vi "LIA_FPGA3a-PD Test-3.vi"() -> (1 "K Constant":fxp<+/-,32,16>, 2 "Nominal Freq":fxp<+/-,64,32>)   [LabVIEW 2012]
uses:
  <vilib>/rvi/DataTransferAndStorage/Container/Common/niFpgaContainerMetaDataKey.ctl
  <vilib>/rvi/DataTransferAndStorage/Container/Common/niFpgaContainerState.ctl
  <vilib>/rvi/DataTransferAndStorage/Container/Common/niFpgaDataTypeControl.ctl
  <vilib>/rvi/DataTransferAndStorage/Container/Common/niFpgaContainerImplementationControl.ctl
  <vilib>/rvi/DataTransferAndStorage/Container/Common/niFpgaContainerArbitrationOptionsControl.ctl
  <vilib>/rvi/DataTransferAndStorage/Container/Common/niFpgaTransferTypeControl.ctl
  <vilib>/rvi/DataTransferAndStorage/Container/Common/niFpgaContainerInitializationParameters.ctl
  <vilib>/rvi/Memory/Memory_Types/niFpgaMemoryInterfaceConfiguration.ctl
  <vilib>/rvi/FIFO/Fifo_Types/niFpgaFifoControlLogicControl.ctl
  <vilib>/Platform/TimedLoop/XDataNode/timing_clust.ctl
  <vilib>/Platform/TimedLoop/XDataNode/nitl_modes.ctl
  <vilib>/Platform/TimedLoop/XDataNode/wakeup.ctl
  <vilib>/rvi/FXPMathLib/FxpSinAndCos/subVIs/nifxpmath_SinAndCos_SimConfig.ctl
  <vilib>/rvi/FXPMathLib/basic elements/FxpIntAccumulator/subVIs/nifxpmath_IntAccumulator_SimConfig.ctl
  <vilib>/rvi/DataTransferAndStorage/Container/Common/niFpgaContainerGetUniqueNameForEmu.vi
  <vilib>/rvi/DataTransferAndStorage/Container/Common/niFpgaContainerSetEmuInfo.vi
  <vilib>/rvi/eio/common/nirviEmuReportErrorAndStop.vi
  <vilib>/rvi/FXPMathLib/FxpSinAndCos/simVIs/DllFxpSinAndCosTemp_sub.vi
  <vilib>/rvi/FXPMathLib/basic elements/FxpIntAccumulator/simVIs/DllFxpIntAccumulator_sub.vi
  <vilib>/rvi/eio/common/nirviEmuTemplateMethod_errors.vi
  <vilib>/rvi/Emulation/niFpgaSctlEmulationGetInTimedLoop.vi
  <vilib>/rvi/FIFO/Fifo_Resource/nirvififoEmulationSetSize.vi
  <vilib>/rvi/errors/niFpgaSetErrorForExecOnDevCompSimple.vi
  <vilib>/rvi/Emulation/niFpgaSctlEmulationFifoFullMgr.vi
  <vilib>/rvi/Emulation/niFpgaSctlEmulationResourceMgr.vi
  <vilib>/rvi/Emulation/niFpgaSctlEmulationRegisterWithScheduler.vi
  <vilib>/rvi/Emulation/niFpgaSctlEmulationScheduler.vi
  <vilib>/rvi/LocalResourceManager/LocalResourceManager.xnode
  <vilib>/Platform/TimedLoop/XDataNode/XDataNode.xnode
  <vilib>/rvi/FXPMathLib/FxpSinAndCos/XNode/nifxpmath_SinAndCos.xnode
  <vilib>/rvi/FXPMathLib/basic elements/FxpIntAccumulator/XNode/nifxpmath_IntAccumulator.xnode
  <vilib>/rvi/FXPMathLib/FxpInterpret/XNode/nifxpmath_Interpret.xnode
  <vilib>/eio/EIONode/EIONode.xnode
  <vilib>/rvi/DataTransferAndStorage/Container/XNode/niFpgaContainer.xnode
  <vilib>/rvi/FIFO/Fifo_Resource/nirvififoEmulationWrite.vi
  <vilib>/rvi/FIFO/Fifo_Resource/nirvififoEmulationRead.vi
  <vilib>/Platform/TimedLoop/XDataNode/XDNodeRunTimeDep.lvlib
panel:
  out "Test Input":fxp<+/-,64,32>
  out "Sine Output":fxp<+/-,64,32>
  in  "Voltage (V)":fxp<+,64,12>=3276.8125
  in  "Z":fxp<+/-,64,16>
  out "Summation":fxp<+/-,64,32>
  out "Radians":fxp<+/-,14,5>
  out "Cos":fxp<+/-,14,2>
  out "Sin":fxp<+/-,14,2>
  in  "Period":u16=1000
  out "ticks":u16
  out "ref":i16 format="%.0x"
  out "sig":i16 format="%.0x"
  out "channelQ":i64
  out "channelI":i64
  out "f":fxp<+/-,32,0> format="%.32g"
  in  "start":bool
  in  "dec2":i16=1
  in  "K":fxp<+,16,0>=0.001007080078125
  in  "nominal freq":fxp<+,16,0>=0.010009765625
  in  "dec1":i16=1
  in  "stages":i8=1
  in  "stop":bool
  in  "decimation":i16=1024
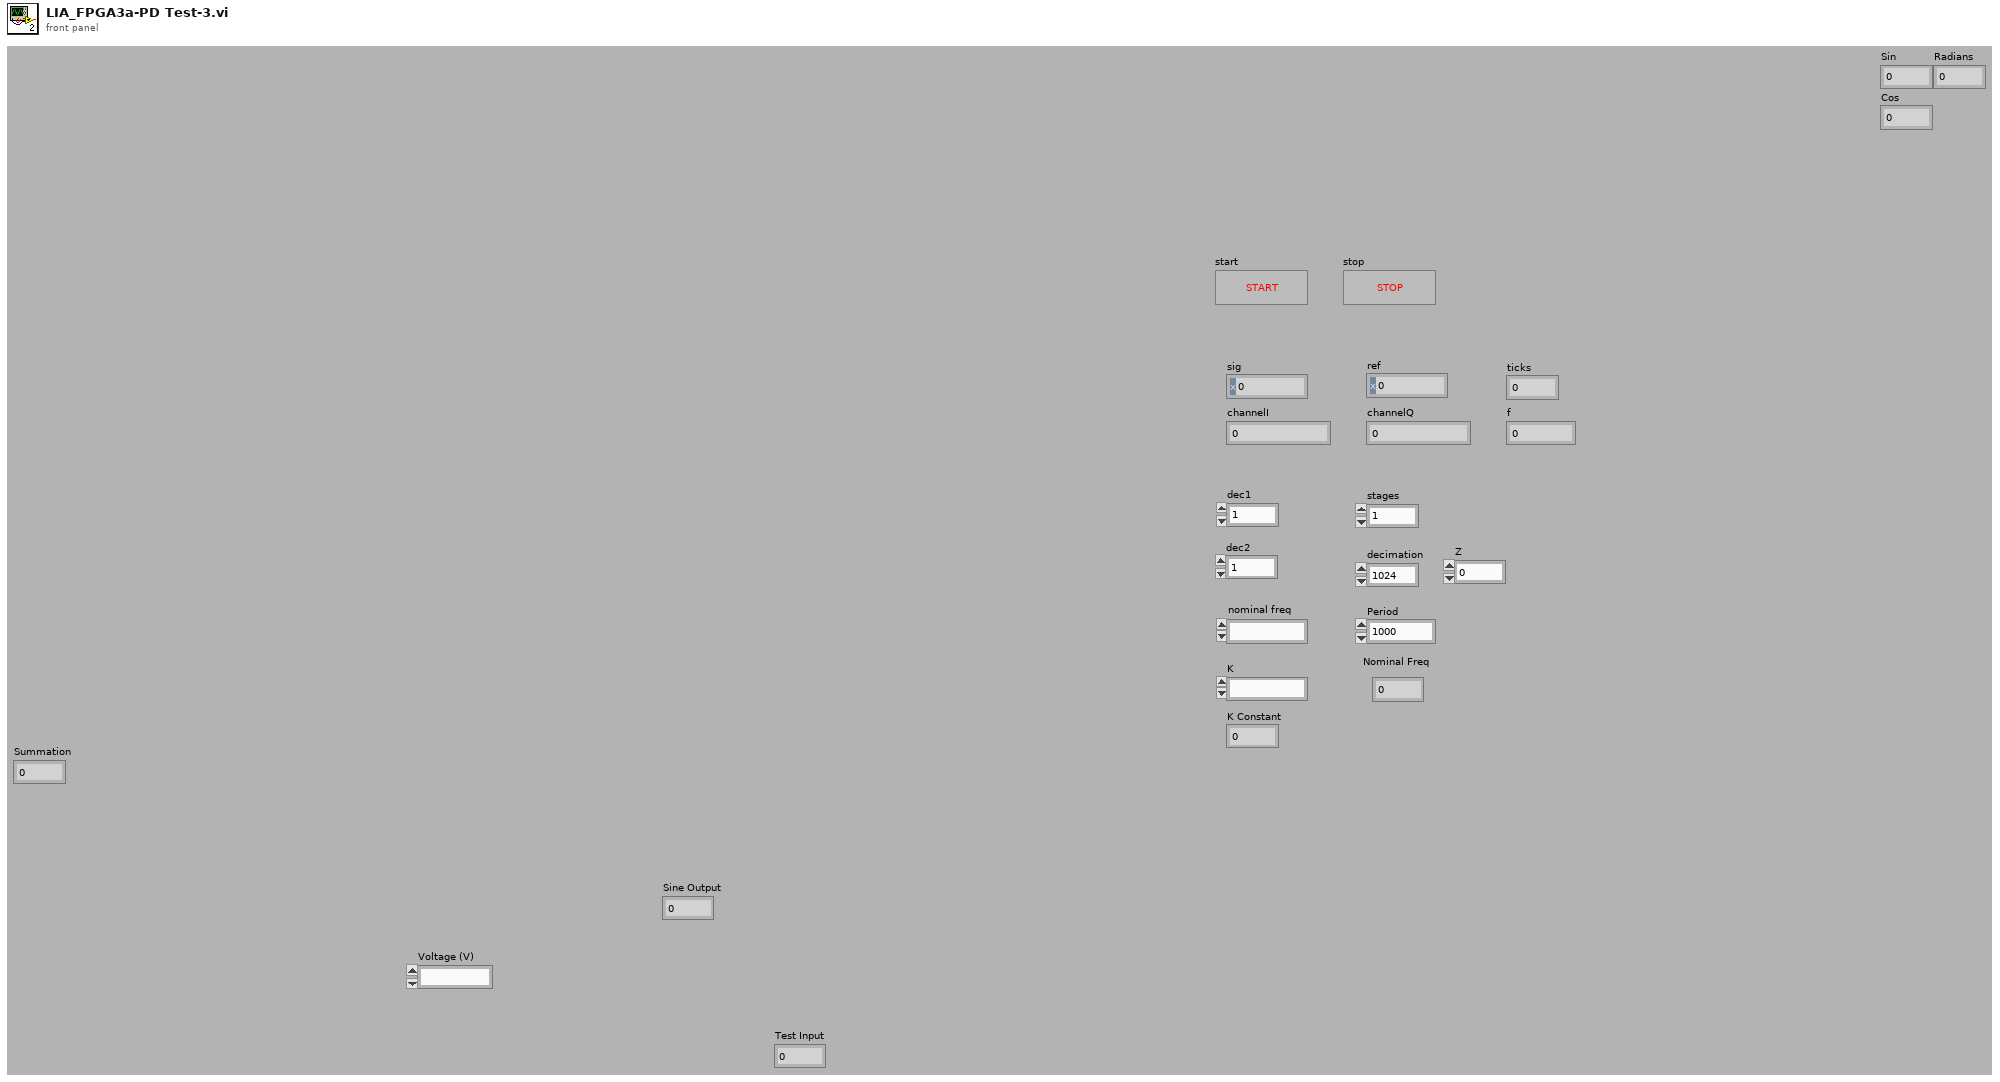
[diagram p1: front panel]
types:
  T1 = typedef "XDNodeRunTimeDep.lvlib/timing_clust.ctl" = cluster{"Expected End [f-1]":u64, "Actual End [f-1]":u64, "Finished Late? [f-1]":bool, "Expected End [i-1]":u64, "Actual End [i-1]":u64, "Finished Late? [i-1]":bool, "Expected Start [i]":u64, "Actual Start [i]":u64, "Expected Start [f]":u64, "Actual Start [f]":u64, "Source Name":string, "Structure Name":string, "Period":i64, "Deadline":i64, "Offset":i64, "Start":i64, "Priority":i32, "Timeout":i32, "Mode":T2, "Wakeup Reason":T3, "Error":errorcluster, "Source Type":string, "Secondary Source Type":string, "Global End Time":u64, "Global Start Time":u64, "Frame Duration":u64, "Iteration Duration":u64, "Assigned CPU":i32, "I/O Scan Engine Mode":u32}
  T2 = typedef "XDNodeRunTimeDep.lvlib/nitl_modes.ctl" = enum32{"No Change", "Process missed periods, maintain original phase", "Discard missed periods, maintain original phase", "Process missed periods, ignore original phase", "Discard missed periods, ignore original phase"}
  T3 = typedef "XDNodeRunTimeDep.lvlib/wakeup.ctl" = enum32{"Normal", "Aborted", "Asynchronous wakeup", "Timing source error", "Timed loop error", "Timeout"}
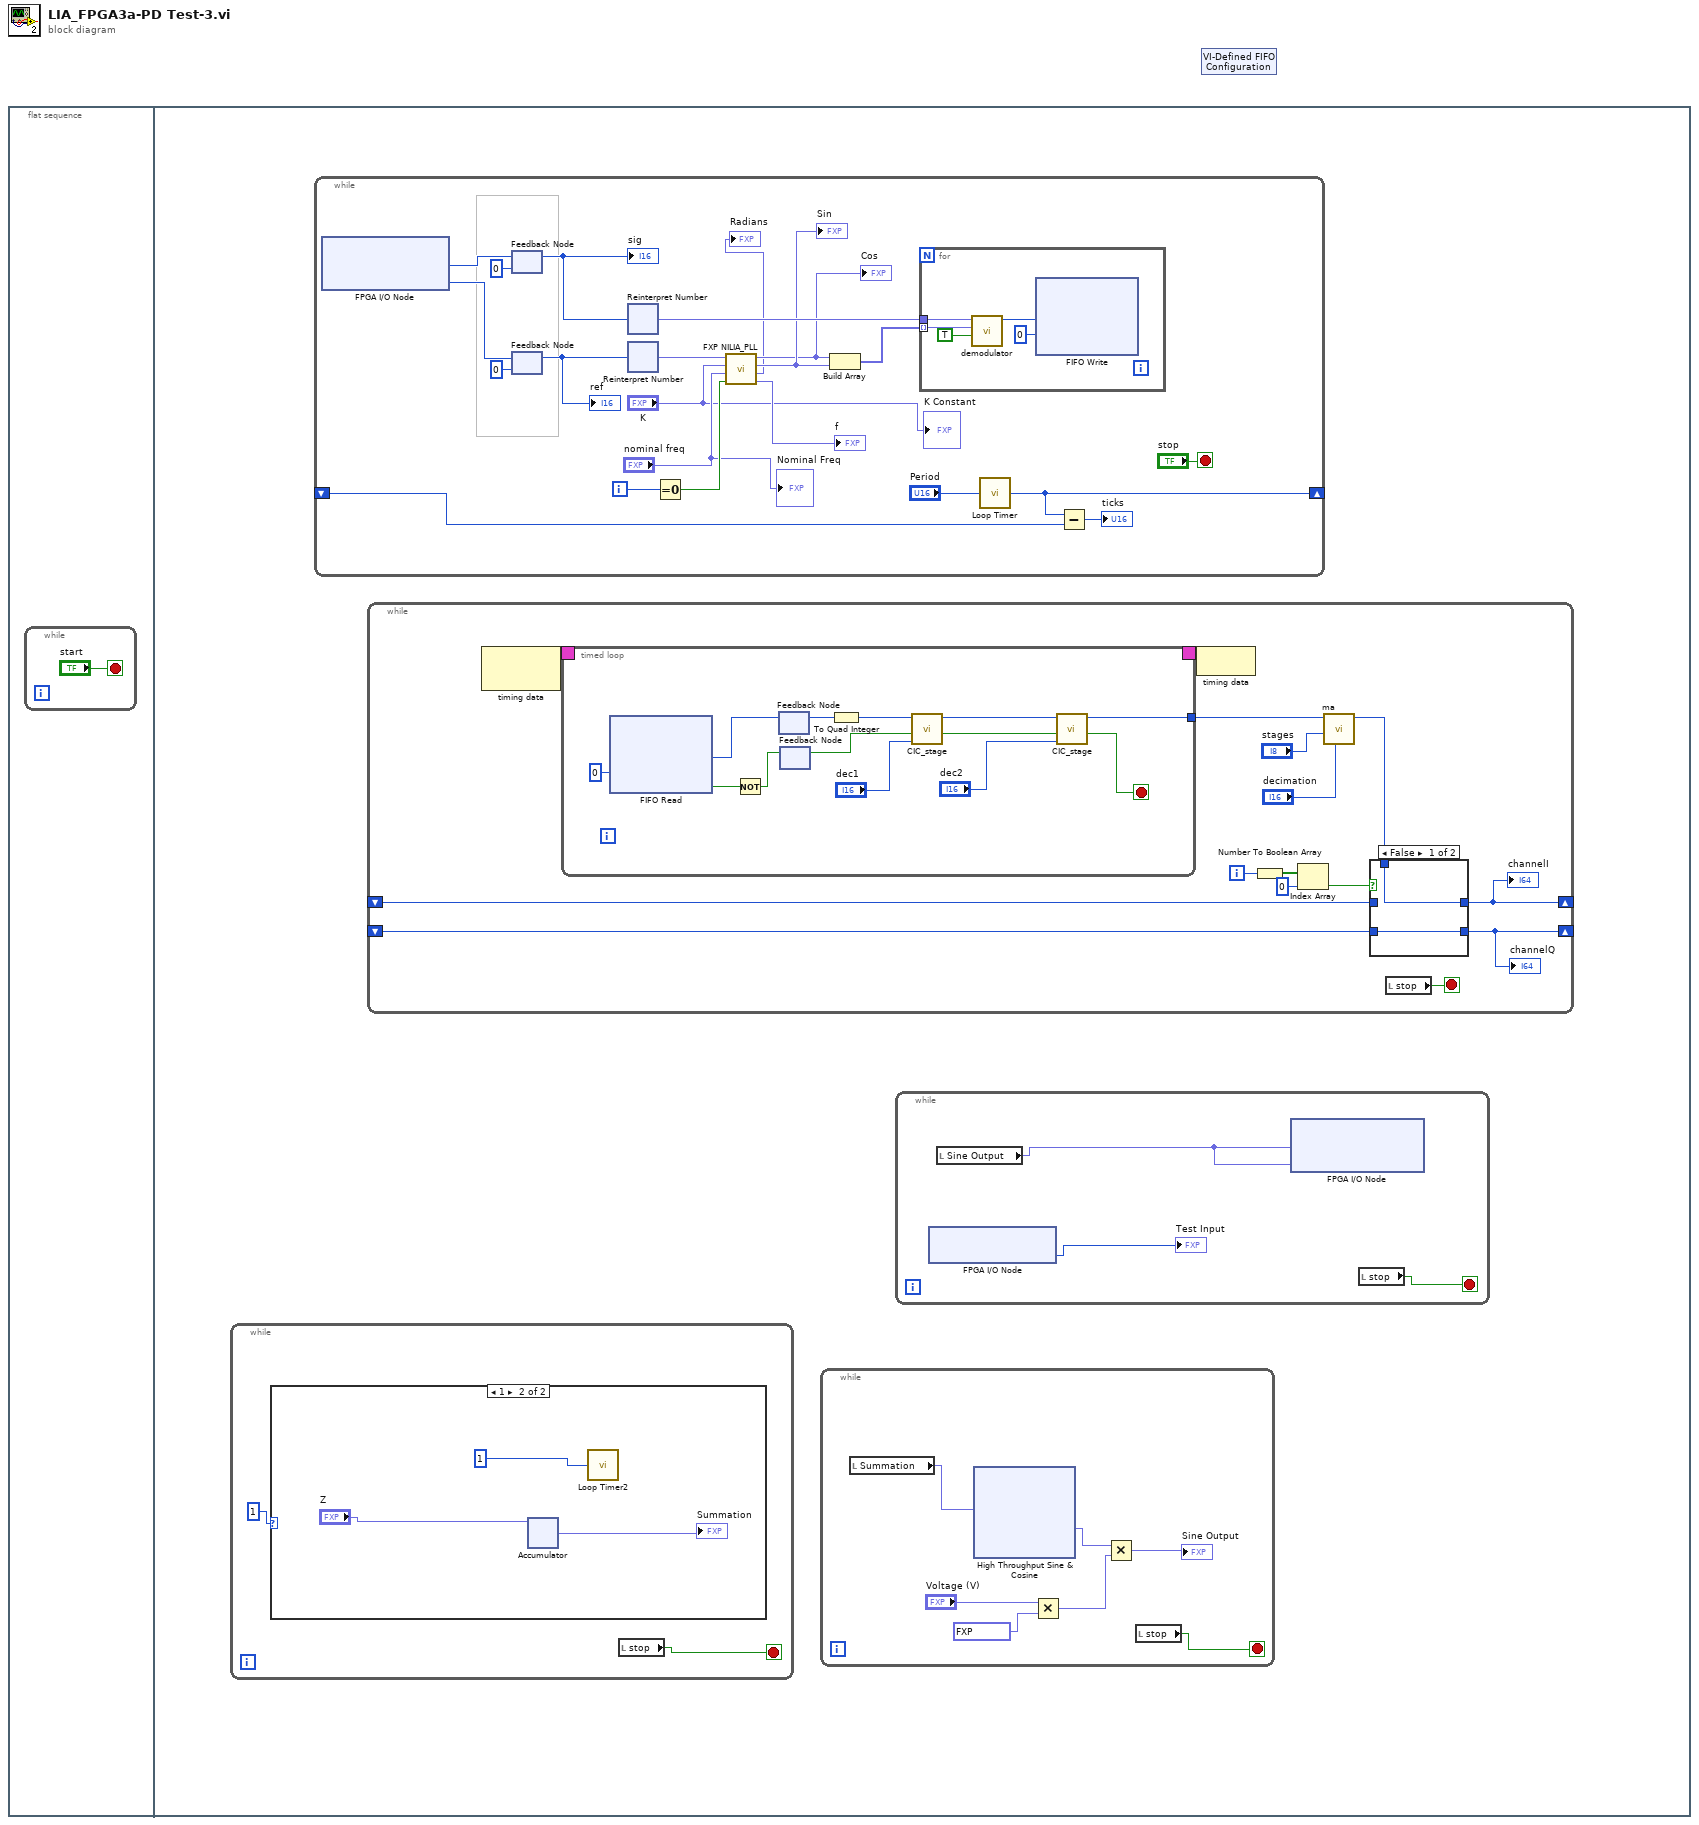
[diagram p0: block diagram]
diagram:
  n1 = flat-sequence {
    frame #0 {
      n2 = while {
        stop <- "start" stop-if-true
      }
    }
    frame #1 {
      n3 = while {
        stop <- w42 stop-if-true
        n4 = case shown="1" 1 {
          frame 0, Default {
          }
          frame 1 {
            n5 = xnode "Accumulator"("x"="Z") -> ("s"=→"Summation":fxp<+/-,64,16>)  [unwired: 4 in, 1 out]
            n6 = call "Loop Timer2"("Count(uSec)"=1) -> ()  [unwired: 1 out]
          }
        }
        n7 = local read "stop"() -> (w42:bool)
      }
      n8 = while {
        shift-right: [w92] -> _
        shift-left: _ -> [w91]
        i -> [w95]
        stop <- "stop" stop-if-true
        n9 = xnode "FPGA I/O Node"() -> ("Connector0/AI6"=w85:i16, "Connector0/AI7"=w82:i16)  [unwired: 2 in, 2 out]
        n10 = feedback #1(i16 0 ("y")) -> (w84:i16)
        "sig" <- w84
        n11 = feedback-in #1(w85) -> ()
        n12 = feedback #2(i16 0 ("z [I32.1]")) -> (w83:i16)
        "ref" <- w83
        n13 = feedback-in #2(w82) -> ()
        n14 = xnode "Reinterpret Number"("x"=w84) -> ("y"=w88:fxp<+/-,16,1>)
        n15 = xnode "Reinterpret Number"("x"=w83) -> ("y"=w81:fxp<+/-,16,1>)
        n16 = Equal To 0?(x=w95) -> (x = 0?=w79:bool)
        n17 = call "FXP NILIA_PLL.vi"("reset?"=w79, "norminal freq [U16.0]"="nominal freq", "alpha [U16.0]"="K", "x[I16.1]"=w81) -> ("f"=→"f":fxp<+/-,32,0>, "z [I32.1]"=→"Radians":fxp<+/-,32,1>, "sin(z)"=w76:fxp<+/-,16,2>, "cos(z)"=w75:fxp<+/-,16,2>)  [unwired: 4 in]
        "Sin" <- w76
        "Cos" <- w75
        n18 = Build Array(w75, w76) -> (w89:fxp<+/-,16,2>[])
        n19 = for {
          tunnel: w88 -> [w98]
          tunnel: w89 -> [w96] mode=indexing
          n20 = call "demodulator.vi"("New Data"=TRUE, "ref"=w96, "signal"=w98) -> ("x*y"=w99:i32)  [unwired: 8 out]
          n21 = xnode ("FIFO Write")("Element"=w99, "Timeout"=0) -> ()  [unwired: 1 in, 2 out]
        }
        n22 = call "Loop Timer"("Count(Ticks)"="Period") -> ("Tick Count(Ticks)"=w92:u16)
        n23 = Subtract(x=w92, y=w91) -> (x-y=→"ticks":u16)
        "Nominal Freq" <- "nominal freq"
        "K Constant" <- "K"
      }
      n24 = while {
        shift-right: [w102] -> _
        shift-left: _ -> [w104]
        shift-right: [w101] -> _
        shift-left: _ -> [w103]
        i -> [w109]
        stop <- w111 stop-if-true
        n25 = node-c288() -> (w115:T1)  [unwired: 1 out]
        n26 = timed-loop {
          timing: w115 -> [_]
          timing-out: [_] -> w114
          tunnel: [w123] -> w110
          stop <- w122 stop-if-true
          n27 = xnode ("FIFO Read")("Timeout"=0) -> ("Element"=w130:i32, "Timed Out?"=w129:bool)  [unwired: 1 in, 1 out]
          n28 = Not(x=w129) -> (.not. x?=w128:bool)
          n29 = feedback-in #3(w130) -> ()
          n30 = feedback #3() -> (w132:i32)  [unwired: 1 out]
          n31 = feedback-in #4(w128) -> ()
          n32 = feedback #4() -> (w126:bool)  [unwired: 1 out]
          n33 = To Quad Integer(1:w132) -> (0:w127:i64)
          n34 = call "CIC_stage.vi"("decimate factor"="dec1", "New Data"=w126, "input"=w127) -> ("Data Ready"=w124:bool, "output"=w125:i64)  [unwired: 7 out]
          n35 = call "CIC_stage.vi"("decimate factor"="dec2", "New Data"=w124, "input"=w125) -> ("Data Ready"=w122:bool, "output"=w123:i64)  [unwired: 7 out]
        }
        n36 = node-c288(w114) -> ()
        n37 = Number To Boolean Array(number=w109) -> (Boolean array=w108:bool[])
        n38 = Index Array "Index Array"(array=w108, index=0) -> (element=w106:bool)
        n39 = call "ma.vi"("decimate"="decimation", "stages"="stages", "input"=w110) -> ("output"=w105:i64)  [unwired: 8 out]
        n40 = case shown="False" w106 {
          tunnel: w105 -> [w117 w119]
          tunnel: [w117 w118] -> w102
          tunnel: [w116 w119] -> w101
          tunnel: w104 -> [_ w118]
          tunnel: w103 -> [w116 _]
          frame False {
          }
          frame True {
          }
        }
        "channelI" <- w102
        "channelQ" <- w101
        n41 = local read "stop"() -> (w111:bool)
      }
      n42 = while {
        stop <- w5 stop-if-true
        n43 = local read "Summation"() -> (w11:fxp<+/-,64,32>)
        n44 = xnode "High Throughput Sine & Cosine"("x (pi)"=w11) -> ("sin(x)"=w10:fxp<+/-,16,2>)  [unwired: 1 out]
        n45 = Multiply(x="Voltage (V)", y=fxp<+,17,12> 3276.8125) -> (x*y=w6:fxp<+,64,24>)
        n46 = Multiply(x=w10, y=w6) -> (x*y=→"Sine Output":fxp<+/-,64,26>)
        n47 = local read "stop"() -> (w5:bool)
      }
      n48 = while {
        stop <- w3 stop-if-true
        n49 = xnode "FPGA I/O Node"() -> ("Connector0/AI5"=→"Test Input":i16)  [unwired: 1 in, 1 out]
        n50 = local read "Sine Output"() -> (w2:fxp<+/-,64,32>)
        n51 = xnode "FPGA I/O Node"("Connector0/AO2"=w2, "Connector0/AO1"=w2) -> ()  [unwired: 2 in, 2 out]
        n52 = local read "stop"() -> (w3:bool)
      }
    }
  }
  n53 = xnode "VI-Defined FIFO Configuration"() -> ()  [unwired: 1 out]
